vi "Disable Tab Control_LV2012_NI Verified.vi"() -> ()   [LabVIEW 2012]
doc: "This VI demonstrates several VI Server properties of Tab controls. It shows how to enable/disable a specific\npage of the tab control and how to programmatically toggle between pages."
uses:
  Controls/States.ctl
panel:
  in  "Tab Control":enum32{"Parameters", "Results"}(tab)
  in  "Submit":bool
  in  "Standard Deviation":dbl(knob)=0.7039150787906233 scale=0.0..10.0
  in  "Sine Amplitude":dbl=7.0
  in  "Ramp Control End":dbl=3.0
  in  "Ramp Control Start":dbl=6.0
  out "Test Results":dbl[][](graph)
  in  "stop":bool
  # "Overview: This example demonstrates several VI Server properties of Tab controls. It shows how to enable/disable a specific\npage of the tab control and how to programmatically toggle between pages.\nRequirements: LabVIEW 2012 or compatible\nInstructions:\n1- Run this VI\n2- Enter your configuration on Parameters Tab & click Submit\n3- Check Results and click on Finished."
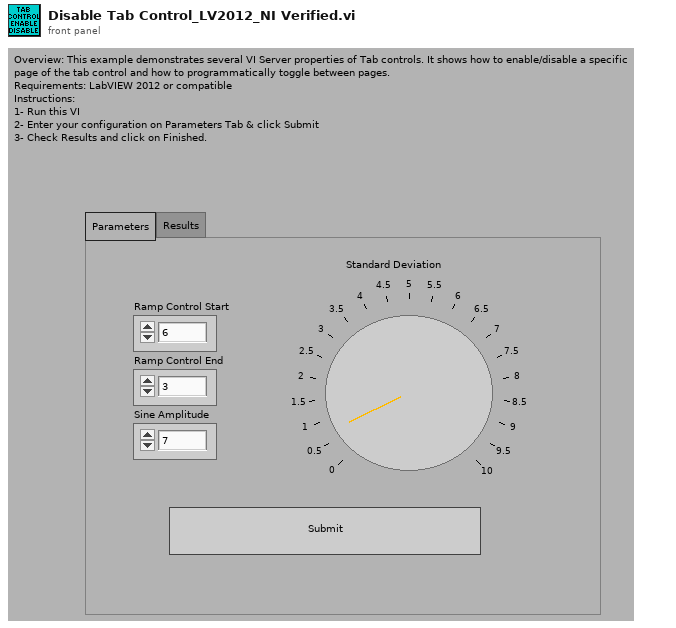
[diagram p1: front panel]
types:
  T1 = typedef "States.ctl" = enum16{"Acquire", "Process", "Display", "Quit"}
  T2 = enum32{"Page Enabled", "Page Disabled", "Page Disabled & Grayed"}
  T3 = cluster{"Ramp Control Start":dbl, "Ramp Control End":dbl, "Sine Amplitude":dbl, "Standard Deviation":dbl}
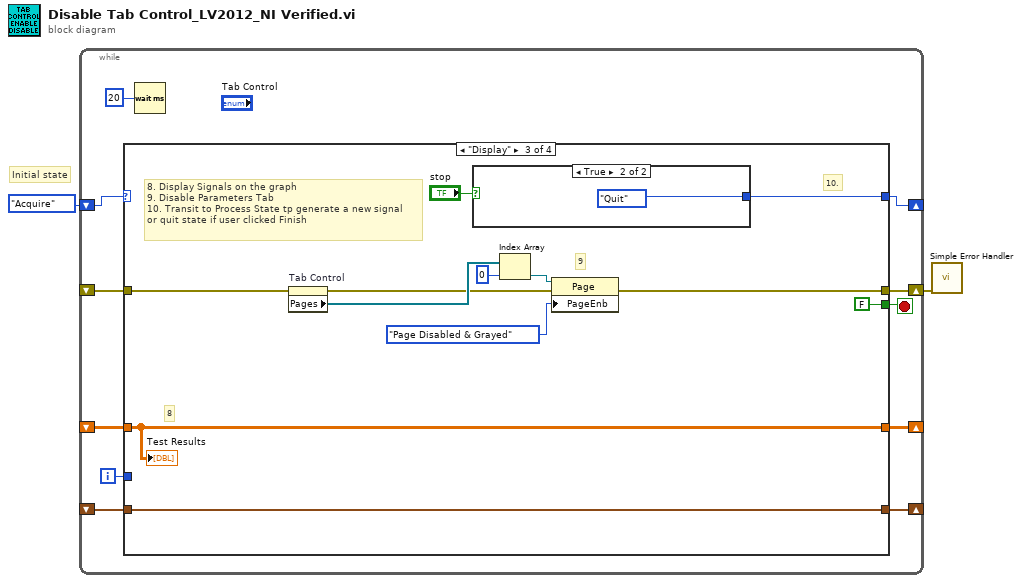
[diagram p0: block diagram]
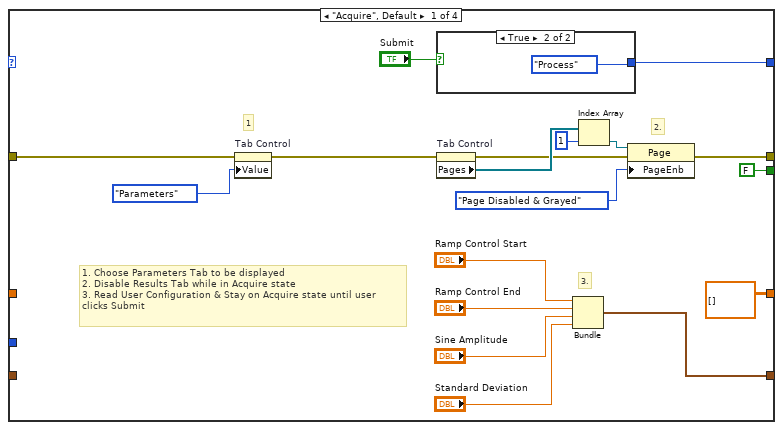
[diagram p2: hidden frame]
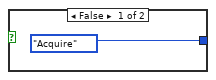
[diagram p3: hidden frame]
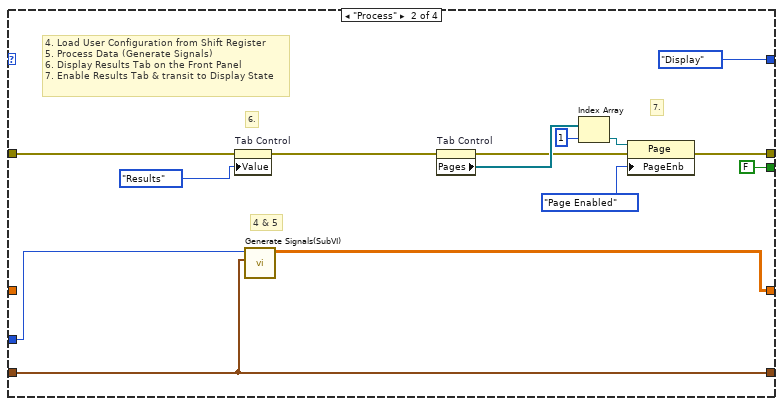
[diagram p4: hidden frame]
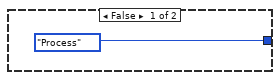
[diagram p5: hidden frame]
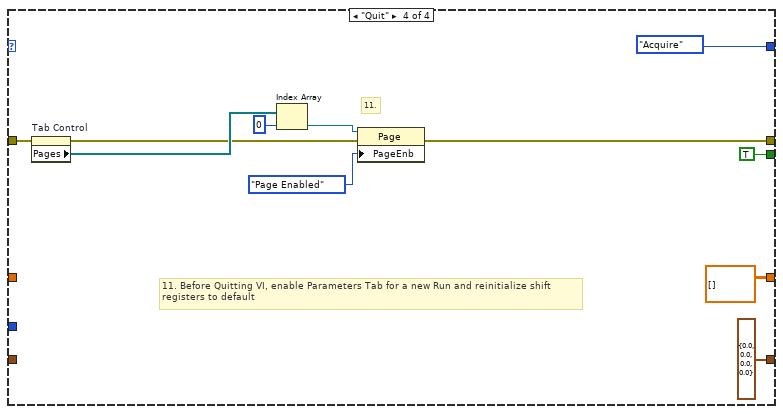
[diagram p6: hidden frame]
diagram:
  # "Initial state"
  n1 = while {
    shift-right: [w11] -> _
    shift-left: States."Acquire" -> [w12]
    shift-right: [w10] -> _
    shift-left: _ -> [w9]
    shift-right: [w7] -> w1
    shift-left: _ -> [w6]
    shift-right: [w4] -> _
    shift-left: _ -> [w3]
    i -> [w5]
    stop <- w8 stop-if-true
    n2 = case shown="\"Display\"" w12 {
      tunnel: [w31 States."Display" w57 States."Acquire"] -> w11
      tunnel: [dbl[][] [] w47 w59 dbl[][] []] -> w10
      tunnel: w9 -> [_ _ w59 _]
      tunnel: [FALSE FALSE FALSE TRUE] -> w8
      tunnel: [w26 w39 w50 w65] -> w7
      tunnel: w6 -> [w22 w45 w51 w66]
      tunnel: w5 -> [_ w38 _ _]
      tunnel: [w16 w37 w49 T3 {"Ramp Control Start"=0.0, "Ramp Control End"=0.0, "Sine Amplitude"=0.0, "Standard Deviation"=0.0}] -> w4
      tunnel: w3 -> [_ w37 w49 _]
      frame "Acquire", Default {
        # "3."
        # "1"
        # "2."
        # "1. Choose Parameters Tab to be displayed\n2. Disable Results Tab while in Acquire state\n3. Read User Configuration & Stay on Acquire state until user \nclicks Submit"
        n3 = property on="Tab Control" class="TabCtl (strict)"(error in=w22, "Value"=enum32{"Parameters", "Results"}."Parameters" ("Tab Control")) -> (error out=w21:errorcluster)  [unwired: 1 in, 1 out]
        n4 = case shown="True" "Submit" {
          tunnel: [States."Acquire" States."Process"] -> w31
          frame False {
          }
          frame True {
          }
        }
        n5 = property on="Tab Control" class="TabCtl (strict)"(error in=w21) -> (error out=w23:errorcluster, "Pages"=w27:refnum<vi>[])  [unwired: 1 in, 1 out]
        n6 = Bundle("Ramp Control Start"="Ramp Control Start", "Ramp Control End"="Ramp Control End", "Sine Amplitude"="Sine Amplitude", "Standard Deviation"="Standard Deviation") -> (w16:T3)  [unwired: 1 in]
        n7 = Index Array(array=w27, index=1) -> (element=w25:refnum<vi>)
        n8 = property class="Page"(reference=w25, error in=w23, "PageEnb"=T2."Page Disabled & Grayed" ("Page Enabled State")) -> (error out=w26:errorcluster)  [unwired: 1 out]
      }
      frame "Process" {
        # "4 & 5"
        # "4. Load User Configuration from Shift Register\n5. Process Data (Generate Signals)\n6. Display Results Tab on the Front Panel\n7. Enable Results Tab & transit to Display State"
        # "7."
        # "6."
        n9 = property on="Tab Control" class="TabCtl (strict)"(error in=w45, "Value"=enum32{"Parameters", "Results"}."Results" ("Tab Control")) -> (error out=w40:errorcluster)  [unwired: 1 in, 1 out]
        n10 = call "Generate Signals(SubVI).vi"("Input Parameters"=w37, "Sample Index"=w38) -> ("Data Out"=w47:dbl[][])  [unwired: 9 in]
        n11 = property on="Tab Control" class="TabCtl (strict)"(error in=w40) -> (error out=w41:errorcluster, "Pages"=w44:refnum<vi>[])  [unwired: 1 in, 1 out]
        n12 = Index Array(array=w44, index=1) -> (element=w43:refnum<vi>)
        n13 = property class="Page"(reference=w43, error in=w41, "PageEnb"=T2."Page Enabled" ("Page Enabled State")) -> (error out=w39:errorcluster)  [unwired: 1 out]
      }
      frame "Display" {
        # "10."
        # "8. Display Signals on the graph\n9. Disable Parameters Tab\n10. Transit to Process State tp generate a new signal \nor quit state if user clicked Finish"
        # "9"
        # "8"
        n14 = property on="Tab Control" class="TabCtl (strict)"(error in=w51) -> (error out=w52:errorcluster, "Pages"=w55:refnum<vi>[])  [unwired: 1 in, 1 out]
        n15 = case shown="True" "stop" {
          tunnel: [States."Process" States."Quit"] -> w57
          frame False {
          }
          frame True {
          }
        }
        n16 = Index Array(array=w55, index=0) -> (element=w54:refnum<vi>)
        n17 = property class="Page"(reference=w54, error in=w52, "PageEnb"=T2."Page Disabled & Grayed" ("Page Enabled State")) -> (error out=w50:errorcluster)  [unwired: 1 out]
        "Test Results" <- w59
      }
      frame "Quit" {
        # "11. Before Quitting VI, enable Parameters Tab for a new Run and reinitialize shift\nregisters to default"
        # "11."
        n18 = property on="Tab Control" class="TabCtl (strict)"(error in=w66) -> (error out=w67:errorcluster, "Pages"=w70:refnum<vi>[])  [unwired: 1 in, 1 out]
        n19 = Index Array(array=w70, index=0) -> (element=w69:refnum<vi>)
        n20 = property class="Page"(reference=w69, error in=w67, "PageEnb"=T2."Page Enabled" ("Page Enabled State")) -> (error out=w65:errorcluster)  [unwired: 1 out]
      }
    }
    n21 = Wait (ms)(milliseconds to wait=u32 20) -> ()  [unwired: 1 out]
  }
  n22 = call <vilib>:"Simple Error Handler.vi"("error in (no error)"=w1) -> ()  [unwired: 4 in, 5 out]
